vi "Read Routing Number.vi"(8 "error in (no error)":errorcluster, 11 "AChecking in":refnum<class "AChecking.lvclass">) -> (0 "error out":errorcluster, 2 "Routing Number":string, 3 "AChecking out":refnum<class "AChecking.lvclass">)   [LabVIEW 2020, in "AChecking.lvclass"]
uses:
  AChecking.lvclass
  AChecking.lvclass/AChecking.ctl
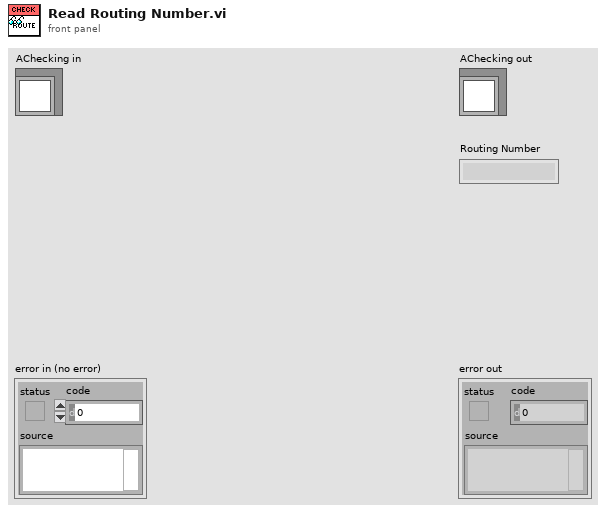
[diagram p1: front panel]
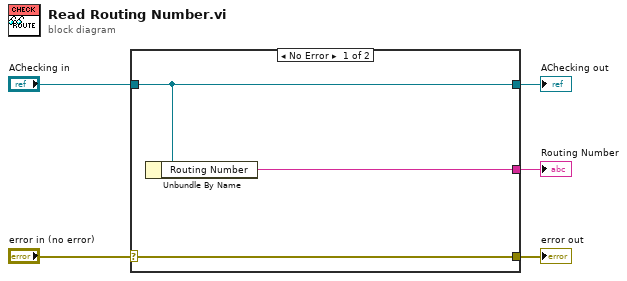
[diagram p0: block diagram]
diagram:
  n1 = case shown="No Error" "error in (no error)" {
    selector: "error in (no error)" -> [w8 w9]
    tunnel: [w8 w9] -> w4
    tunnel: [w7 w10] -> w2
    tunnel: "AChecking in" -> [w7 w10]
    tunnel: [w6 _] -> w1
    frame No Error {
      n2 = Unbundle By Name(w7) -> ("Routing Number"=w6:string)
    }
    frame Error {
    }
  }
  "error out" <- w4
  "AChecking out" <- w2
  "Routing Number" <- w1
